vi "DriveStraightExact.vi"(6 "Angle Wrap":bool, 8 "Start Drive Straight (Hold)":bool=TRUE, 9 "Negates":T4, 10 "PID Constants":T2={"Drive PID"={"proportional gain (Kc)"=1.0, "integral time (Ti, min)"=0.01, "derivative time (Td, min)"=0.0}, "TurnPID"={"proportional gain (Kc)"=1.0, "integral time (Ti, min)"=0.01, "derivative time (Td, min)"=0.0}} {"TurnPID"."derivative time (Td, min)" format="%.3f"; "TurnPID"."integral time (Ti, min)" format="%.3f"; "TurnPID"."proportional gain (Kc)" format="%.3f"; "Drive PID"."derivative time (Td, min)" format="%.3f"; "Drive PID"."integral time (Ti, min)" format="%.3f"; "Drive PID"."proportional gain (Kc)" format="%.3f"}, 11 "Drive Values":T3 {"Throttle Scale" scale=0.0..1.0}) -> (1 "Setpoints":T1, 2 "Cheesy Steer":dbl, 3 "Cheesy Throttle":dbl)   [LabVIEW 2015]
uses:
  <vilib>/addons/control/pid/pid.llb/PID (DBL).vi
  <vilib>/addons/control/pid/NI_PID_pid.lvlib
panel:
  in  "SetpointRef":T1
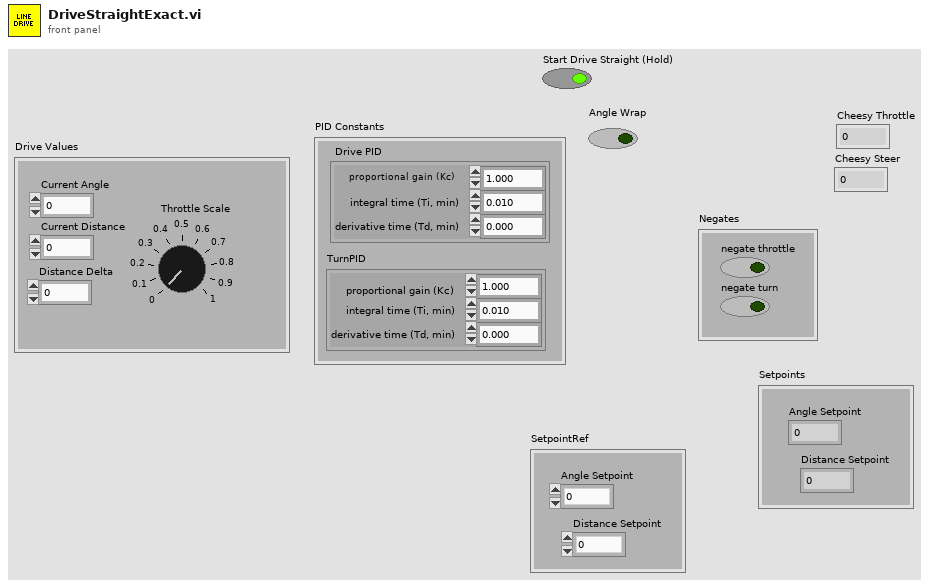
[diagram p1: front panel]
types:
  T1 = cluster{"Angle Setpoint":dbl, "Distance Setpoint":dbl}
  T2 = cluster{"Drive PID":cluster{"proportional gain (Kc)":dbl, "integral time (Ti, min)":dbl, "derivative time (Td, min)":dbl}, "TurnPID":cluster{"proportional gain (Kc)":dbl, "integral time (Ti, min)":dbl, "derivative time (Td, min)":dbl}}
  T3 = cluster{"Distance Delta":dbl, "Throttle Scale":dbl, "Current Angle":dbl, "Current Distance":dbl}
  T4 = cluster{"negate turn":bool, "negate throttle":bool}
  T5 = cluster{"proportional gain (Kc)":dbl, "integral time (Ti, min)":dbl, "derivative time (Td, min)":dbl}
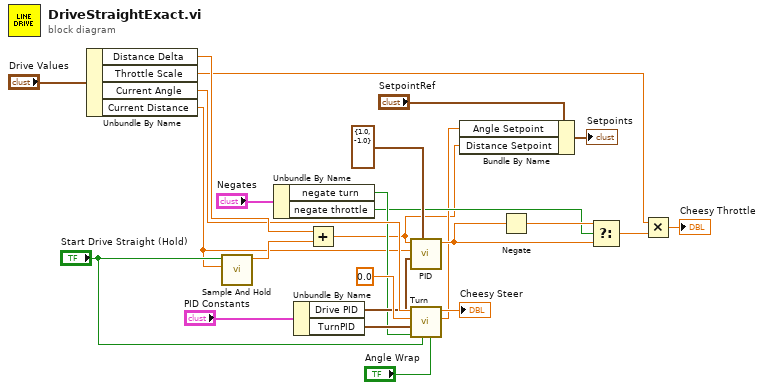
[diagram p0: block diagram]
diagram:
  n1 = Unbundle By Name("Drive Values") -> ("Distance Delta"=w15:dbl, "Throttle Scale"=w14:dbl, "Current Angle"=w13:dbl, "Current Distance"=w6:dbl)
  n2 = call "Sample And Hold.vi"("Signal"=w6, "Condition"="Start Drive Straight (Hold)") -> ("Signal Out"=w23:dbl)  [unwired: 9 in]
  n3 = Unbundle By Name("Negates") -> ("negate turn"=w8:bool, "negate throttle"=w7:bool)
  n4 = Unbundle By Name("PID Constants") -> ("Drive PID"=w10:T5, "TurnPID"=w11:T5)
  n5 = Add(x=w15, y=w23) -> (x+y=w2:dbl)
  n6 = call-poly <vilib>:"PID.vi"("output range"=cluster{"output high":dbl, "output low":dbl} {"output high"=1.0, "output low"=-1.0}, "PID gains"=w10, "process variable"=w6, "setpoint"=w2) -> ("output"=w20:dbl)  [unwired: 6 in, 1 out]
  n7 = call "Turn.vi"("Delta?"="Angle Wrap", "Start Turn"="Start Drive Straight (Hold)", "Negate"=w8, "PID gains"=w11, "Desired Angle"=0.0 ("Delta"), "Current Angle"=w13) -> ("Setpoint"=w3:dbl, "Cheesy Steer"=→"Cheesy Steer":dbl)  [unwired: 3 in, 1 out]
  n8 = Bundle By Name(cluster="SetpointRef", "Angle Setpoint"=w3, "Distance Setpoint"=w2) -> (→"Setpoints":T1)
  n9 = Negate(x=w20) -> (-x=w21:dbl)
  n10 = Select(t=w21, s=w7, f=w20) -> (s? t:f=w18:dbl)
  n11 = Multiply(x=w14, y=w18) -> (x*y=→"Cheesy Throttle":dbl)
